vi "KinectCode.vi"(8 "error in":errorcluster) -> (0 "error out":errorcluster, 3 "HandsApart?":bool)   [LabVIEW 2015]
uses:
  <vilib>/addons/Kinect/Skeleton Vertex Index.ctl
panel:
  out "Distance":sgl
  in  "DistanceVariable":sgl=0.75
  out "HandsTracked?":bool
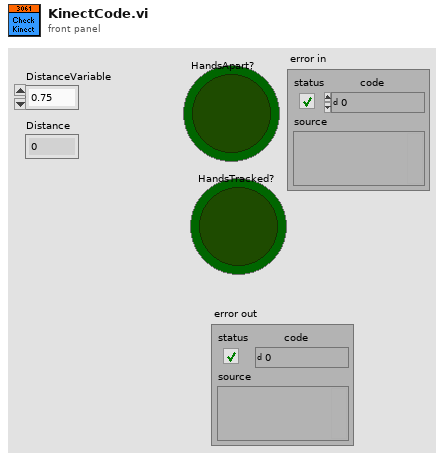
[diagram p1: front panel]
types:
  T1 = typedef "Skeleton Vertex Index.ctl" = i32
  T2 = typedef "SkeletonVertexTrackState.ctl" = enum32{"NotTracked", "Inferred", "Tracked"}
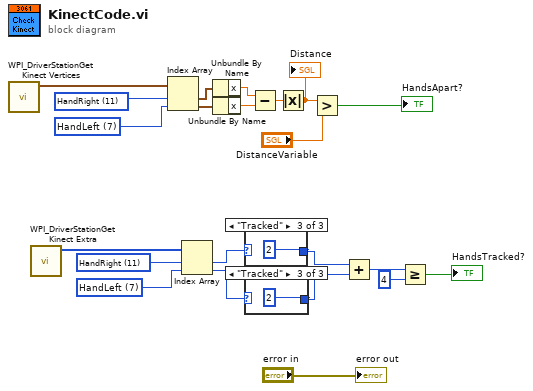
[diagram p0: block diagram]
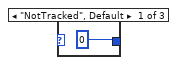
[diagram p2: hidden frame]
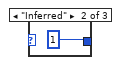
[diagram p3: hidden frame]
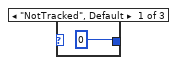
[diagram p4: hidden frame]
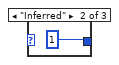
[diagram p5: hidden frame]
diagram:
  w10 = T1 7 items=["HipCenter", "Spine", "ShoulderCenter", "Head", "ShoulderLeft", "ElbowLeft", "WristLeft", "HandLeft", "ShoulderRight", "ElbowRight", "WristRight", "HandRight", "HipLeft", "KneeLeft", "AnkleLeft", "FootLeft", "HipRight", "KneeRight", "AnkleRight", "FootRight"] ("Skeleton Joints")
  w11 = T1 11 items=["HipCenter", "Spine", "ShoulderCenter", "Head", "ShoulderLeft", "ElbowLeft", "WristLeft", "HandLeft", "ShoulderRight", "ElbowRight", "WristRight", "HandRight", "HipLeft", "KneeLeft", "AnkleLeft", "FootLeft", "HipRight", "KneeRight", "AnkleRight", "FootRight"] ("Skeleton Joints")
  w20 = T1 7 items=["HipCenter", "Spine", "ShoulderCenter", "Head", "ShoulderLeft", "ElbowLeft", "WristLeft", "HandLeft", "ShoulderRight", "ElbowRight", "WristRight", "HandRight", "HipLeft", "KneeLeft", "AnkleLeft", "FootLeft", "HipRight", "KneeRight", "AnkleRight", "FootRight"] ("Skeleton Joints")
  w21 = T1 11 items=["HipCenter", "Spine", "ShoulderCenter", "Head", "ShoulderLeft", "ElbowLeft", "WristLeft", "HandLeft", "ShoulderRight", "ElbowRight", "WristRight", "HandRight", "HipLeft", "KneeLeft", "AnkleLeft", "FootLeft", "HipRight", "KneeRight", "AnkleRight", "FootRight"] ("Skeleton Joints")
  n1 = call <vilib>:"WPI_DriverStationGet Kinect Vertices.vi"() -> ("Skeleton Vertices"=w12:cluster{"x":sgl, "y":sgl, "z":sgl}[])  [unwired: 10 in, 1 out]
  n2 = call <vilib>:"WPI_DriverStationGet Kinect Extra.vi"() -> ("Skeleton Tracking State"=w22:T2[])  [unwired: 7 in, 4 out]
  n3 = Index Array(array=w12, index #1=w11, index #2=w10) -> (element #1=w9:cluster{"x":sgl, "y":sgl, "z":sgl}, element #2=w8:cluster{"x":sgl, "y":sgl, "z":sgl})
  n4 = Index Array(array=w22, index #1=w21, index #2=w20) -> (element #1=w18:T2, element #2=w19:T2)
  n5 = Unbundle By Name(w9) -> ("x"=w6:sgl)
  n6 = Unbundle By Name(w8) -> ("x"=w7:sgl)
  n7 = case shown="\"Tracked\"" w18 {
    tunnel: [0 1 2] -> w17
    frame "NotTracked", Default {
    }
    frame "Inferred" {
    }
    frame "Tracked" {
    }
  }
  n8 = case shown="\"Tracked\"" w19 {
    tunnel: [0 1 2] -> w16
    frame "NotTracked", Default {
    }
    frame "Inferred" {
    }
    frame "Tracked" {
    }
  }
  n9 = Subtract(x=w6, y=w7) -> (x-y=w5:sgl)
  n10 = Absolute Value(x=w5) -> (abs(x)=w4:sgl)
  "Distance" <- w4
  n11 = Greater?(x=w4, y="DistanceVariable") -> (0:→"HandsApart?":bool)
  n12 = Add(x=w17, y=w16) -> (x+y=w15:i32)
  n13 = Greater Or Equal?(x=w15, y=4) -> (x >= y?=→"HandsTracked?":bool)
  "error out" <- "error in"
